vi "Rectangle funct ack completion handler.vi"(11 "Destination folder":path) -> ()   [LabVIEW 2017]
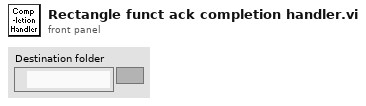
[diagram p1: front panel]
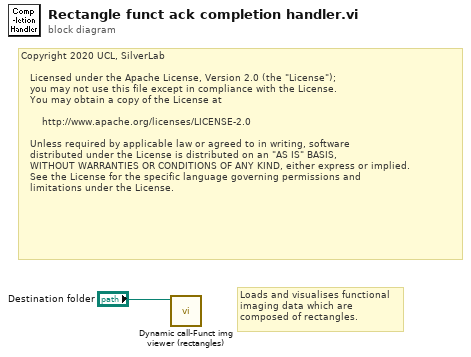
[diagram p0: block diagram]
diagram:
  # "Copyright 2020 UCL, SilverLab\n \n   Licensed under the Apache License, Version 2.0 (the \"License\");\n   you may not use this file except in compliance with the License.\n   You may obtain a copy of the License at\n \n       http://www.apache.org/licenses/LICENSE-2.0\n \n   Unless required by applicable law or agreed to in writing, software\n   distributed under the License is distributed on an \"AS IS\" BASIS,\n   WITHOUT WARRANTIES OR CONDITIONS OF ANY KIND, either express or implied.\n   See the License for the specific language governing permissions and\n   limitations under the License."
  # "Loads and visualises functional imaging data which are composed of rectangles."
  n1 = call "Dynamic call-Funct img viewer (rectangles).vi"("Experiment Path"="Destination folder") -> ()  [unwired: 10 in, 1 out]
